vi "查询历史数据.vi"(10 "日期时间条件":cluster{"年":i32, "月":i32, "周":i32, "日":i32}, 11 "PC个人客户端.lvclass":refnum<class "PC个人客户端.lvclass">) -> (2 "查询结果":T1)   [LabVIEW 2013, in "数据库操作.lvclass"]
panel:
  out "模式":enum16{"年", "月", "周", "日"}(ring)
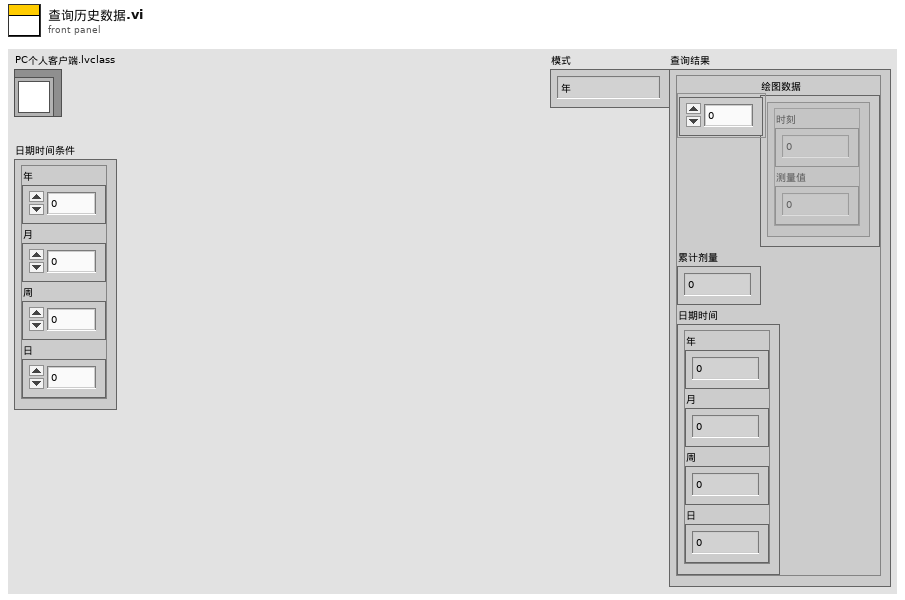
[diagram p1: front panel]
types:
  T1 = cluster{"绘图数据":cluster{"时刻":i32, "测量值":dbl}[], "累计剂量":dbl, "日期时间":cluster{"年":i32, "月":i32, "周":i32, "日":i32}}
  T2 = cluster{"年-条件":string, "月-条件":string, "周-条件":string, "日-条件":string}
  T3 = cluster{"模式":enum16{"年", "月", "周", "日"}, "包括今日？":bool}
  T4 = cluster{"用户名":string, "设备MAC":string, "设备状态":dbl, "密码":string, "职类":dbl, "姓名":string, "电话":string, "邮箱":string, "备注":string, "最后活动":string}
  T5 = typedef "NI_Database_API.lvlib/Conn ObjectReference.ctl" = refnum<k1>
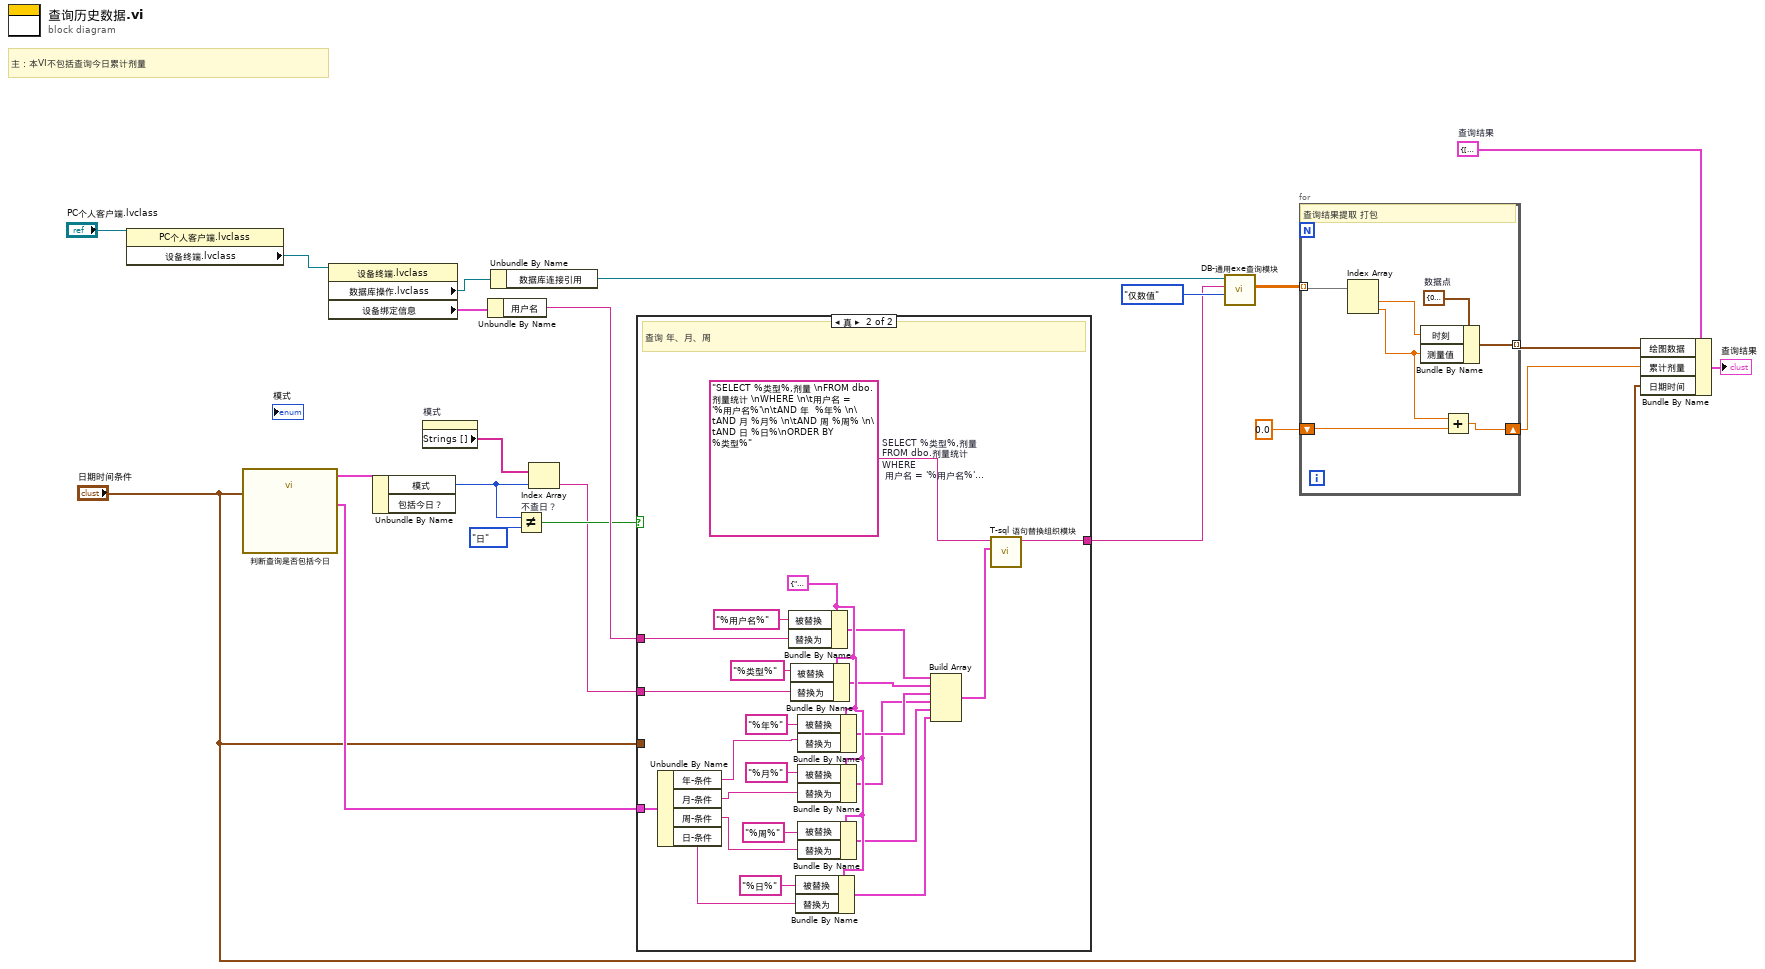
[diagram p0: block diagram]
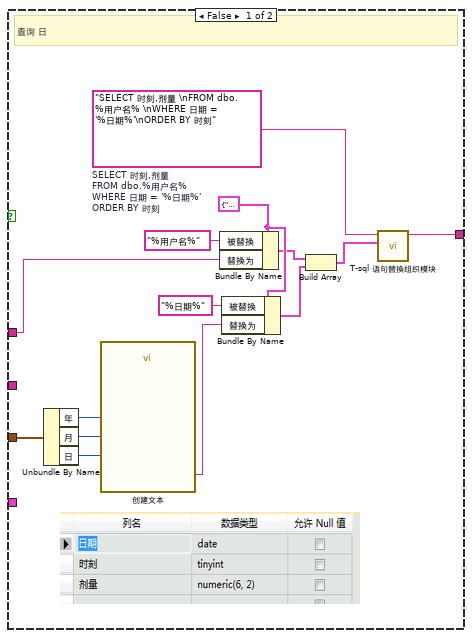
[diagram p2: hidden frame]
diagram:
  w5 = T1 {"绘图数据"=[], "累计剂量"=0.0, "日期时间"={"年"=0, "月"=0, "周"=0, "日"=0}}  # 查询结果
  # "主：本VI不包括查询今日累计剂量"
  n1 = property class="PC个人客户端.lvclass"(reference="PC个人客户端.lvclass") -> ("设备终端.lvclass"=w21:refnum<class "设备终端.lvclass">)  [unwired: 1 in, 2 out]
  n2 = call "判断查询是否包括今日.vi"("日期时间条件"="日期时间条件") -> ("条件语句"=w10:T2, "查询类型"=w19:T3)  [unwired: 9 in]
  n3 = property class="设备终端.lvclass"(reference=w21) -> ("数据库操作.lvclass"=w17:refnum<class "数据库操作.lvclass">, "设备绑定信息"=w20:T4)  [unwired: 1 in, 2 out]
  n4 = Unbundle By Name(w19) -> ("模式"=w13:enum16{"年", "月", "周", "日"})  [unwired: 1 out]
  n5 = property on="模式" class="Enum (严格)"() -> ("Strings []"=w18:string[])  [unwired: 2 in, 2 out]
  n6 = Unbundle By Name(w20) -> ("用户名"=w14:string)
  n7 = Unbundle By Name(w17) -> ("数据库连接引用"=w16:T5)
  n8 = Not Equal? "不查日？"(x=w13, y=enum16{"年", "月", "周", "日"}."日") -> (x != y?=w11:bool)
  n9 = Index Array(array=w18, index=w13) -> (element=w9:string)
  n10 = case shown="真" w11 {
    tunnel: w14 -> [w29 w45]
    tunnel: w10 -> [_ w44]
    tunnel: w9 -> [_ w39]
    tunnel: [w23 w37] -> w8
    tunnel: "日期时间条件" -> [w28 _]
    frame False {
      w35 = cluster{"被替换":string, "替换为":string} {"被替换"="", "替换为"=""} ("替换单元")
      w36 = "SELECT 时刻,剂量 \nFROM dbo.%用户名% \nWHERE 日期 = '%日期%'\nORDER BY 时刻"  # SELECT 时刻,剂量  FROM dbo.%用户名%  WHERE 日期 = '%日期%' ORDER BY 时刻
      # "查询 日"
      n11 = Unbundle By Name(w28) -> ("年"=w27:i32, "月"=w26:i32, "日"=w25:i32)
      n12 = call "创建文本"("年"=w27, "月"=w26, "日"=w25) -> ("Result"=w24:string)  [unwired: 11 in, 1 out]
      n13 = Bundle By Name(cluster=w35, "被替换"="%用户名%", "替换为"=w29) -> (w32:cluster{"被替换":string, "替换为":string})
      n14 = Bundle By Name(cluster=w35, "被替换"="%日期%", "替换为"=w24) -> (w31:cluster{"被替换":string, "替换为":string})
      n15 = Build Array(w32, w31) -> (w30:cluster{"被替换":string, "替换为":string}[])
      n16 = call "T-sql 语句替换组织模块.vi"("替换项"=w30, "T-sql 模板"=w36) -> ("T-sql"=w23:string)  [unwired: 8 in, 1 out]
    }
    frame True {
      w58 = cluster{"被替换":string, "替换为":string} {"被替换"="", "替换为"=""} ("替换单元")
      w59 = "SELECT %类型%,剂量 \nFROM dbo.剂量统计 \nWHERE \n\t用户名 = '%用户名%'\n\tAND 年  %年% \n\tAND 月 %月% \n\tAND 周 %周% \n\tAND 日 %日%\nORDER BY %类型%"  # SELECT %类型%,剂量  FROM dbo.剂量统计  WHERE  	用户名 = '%用户名%' 	AND 年  %年%  	AND 月 %月%  	AND 周 %周%  	AND 日 %日% ORDER BY %类型%
      # "查询 年、月、周"
      n17 = Unbundle By Name(w44) -> ("年-条件"=w43:string, "月-条件"=w42:string, "周-条件"=w41:string, "日-条件"=w40:string)
      n18 = Bundle By Name(cluster=w58, "被替换"="%用户名%", "替换为"=w45) -> (w57:cluster{"被替换":string, "替换为":string})
      n19 = Bundle By Name(cluster=w58, "被替换"="%类型%", "替换为"=w39) -> (w56:cluster{"被替换":string, "替换为":string})
      n20 = Bundle By Name(cluster=w58, "被替换"="%日%", "替换为"=w40) -> (w52:cluster{"被替换":string, "替换为":string})
      n21 = Bundle By Name(cluster=w58, "被替换"="%年%", "替换为"=w43) -> (w55:cluster{"被替换":string, "替换为":string})
      n22 = Bundle By Name(cluster=w58, "被替换"="%月%", "替换为"=w42) -> (w54:cluster{"被替换":string, "替换为":string})
      n23 = Bundle By Name(cluster=w58, "被替换"="%周%", "替换为"=w41) -> (w53:cluster{"被替换":string, "替换为":string})
      n24 = Build Array(w57, w56, w55, w54, w53, w52) -> (w38:cluster{"被替换":string, "替换为":string}[])
      n25 = call "T-sql 语句替换组织模块.vi"("替换项"=w38, "T-sql 模板"=w59) -> ("T-sql"=w37:string)  [unwired: 8 in, 1 out]
    }
  }
  n26 = call "DB-通用exe查询模块.vi"("解析模式"=enum16{"仅数值", "仅字符串", "数值与字符串"}."仅数值", "SQL query"=w8, "数据库连接引用"=w16) -> ("数值数据"=w7:dbl[][])  [unwired: 5 in, 3 out]
  n27 = for {
    tunnel: w7 -> [w66] mode=indexing
    shift-right: [w61] -> w3
    shift-left: 0.0 ("累计剂量") -> [w63]
    tunnel: [w60] -> w4 mode=indexing
    w65 = cluster{"时刻":i32, "测量值":dbl} {"时刻"=0, "测量值"=0.0}  # 数据点
    # "查询结果提取 打包"
    n28 = Index Array(array=w66) -> (element #1=w64:dbl, element #2=w62:dbl)  [unwired: 2 in]
    n29 = Bundle By Name(cluster=w65, "时刻"=w64, "测量值"=w62) -> (w60:cluster{"时刻":i32, "测量值":dbl})
    n30 = Add(x=w62, y=w63) -> (x+y=w61:dbl)
  }
  n31 = Bundle By Name(cluster=w5, "绘图数据"=w4, "累计剂量"=w3, "日期时间"="日期时间条件") -> (→"查询结果":T1)
